vi "ProcessFingers.vi"() -> ()   [LabVIEW 2021]
uses:
  <vilib>/picture/picture.llb/Draw True-Color Pixmap.vi
panel:
  in  "big Or small":i32
  in  "Total Number of Fingers":i32
  in  "range":i32
  out "found fingers":bool
  in  "fingers counter":i32
  out "Little Finger":bool
  out "Ring Finger":bool
  out "Middle Finger":bool
  out "Index Finger":bool
  in  "right counter":i32
  in  "left counter":i32
  in  "j":i32
  in  "i":i32
  in  "bottom counter":i32
  in  "top counter":i32
  in  "thumb counter":i32
  out "Thumb":bool
  out "Right":bool
  out "Left":bool
  out "Black and White Image":picture
  in  "stop":bool
  out "Grayscale Image":picture
  out "Original lmage":picture
  in  "Path":path
  # "Upload Image to be Processed"
  # "Image Data"
  # "Detected Hand"
  # "Detected Fingers"
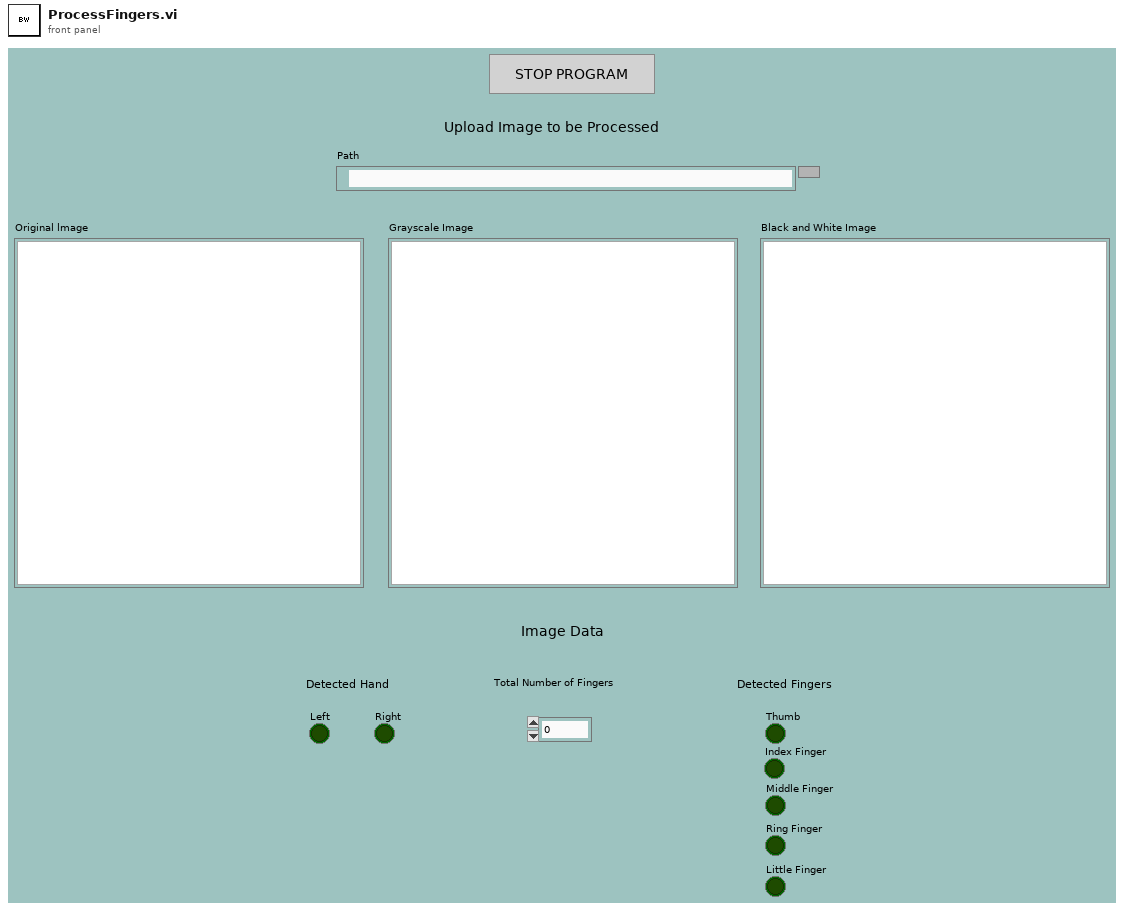
[diagram p1: front panel]
types:
  T1 = typedef "imagedata.ctl" = cluster{"image type":i32, "image depth":i32, "image":u8[], "mask":u8[], "colors":u32[], "Rectangle":cluster{"left":i16, "top":i16, "right":i16, "bottom":i16}}
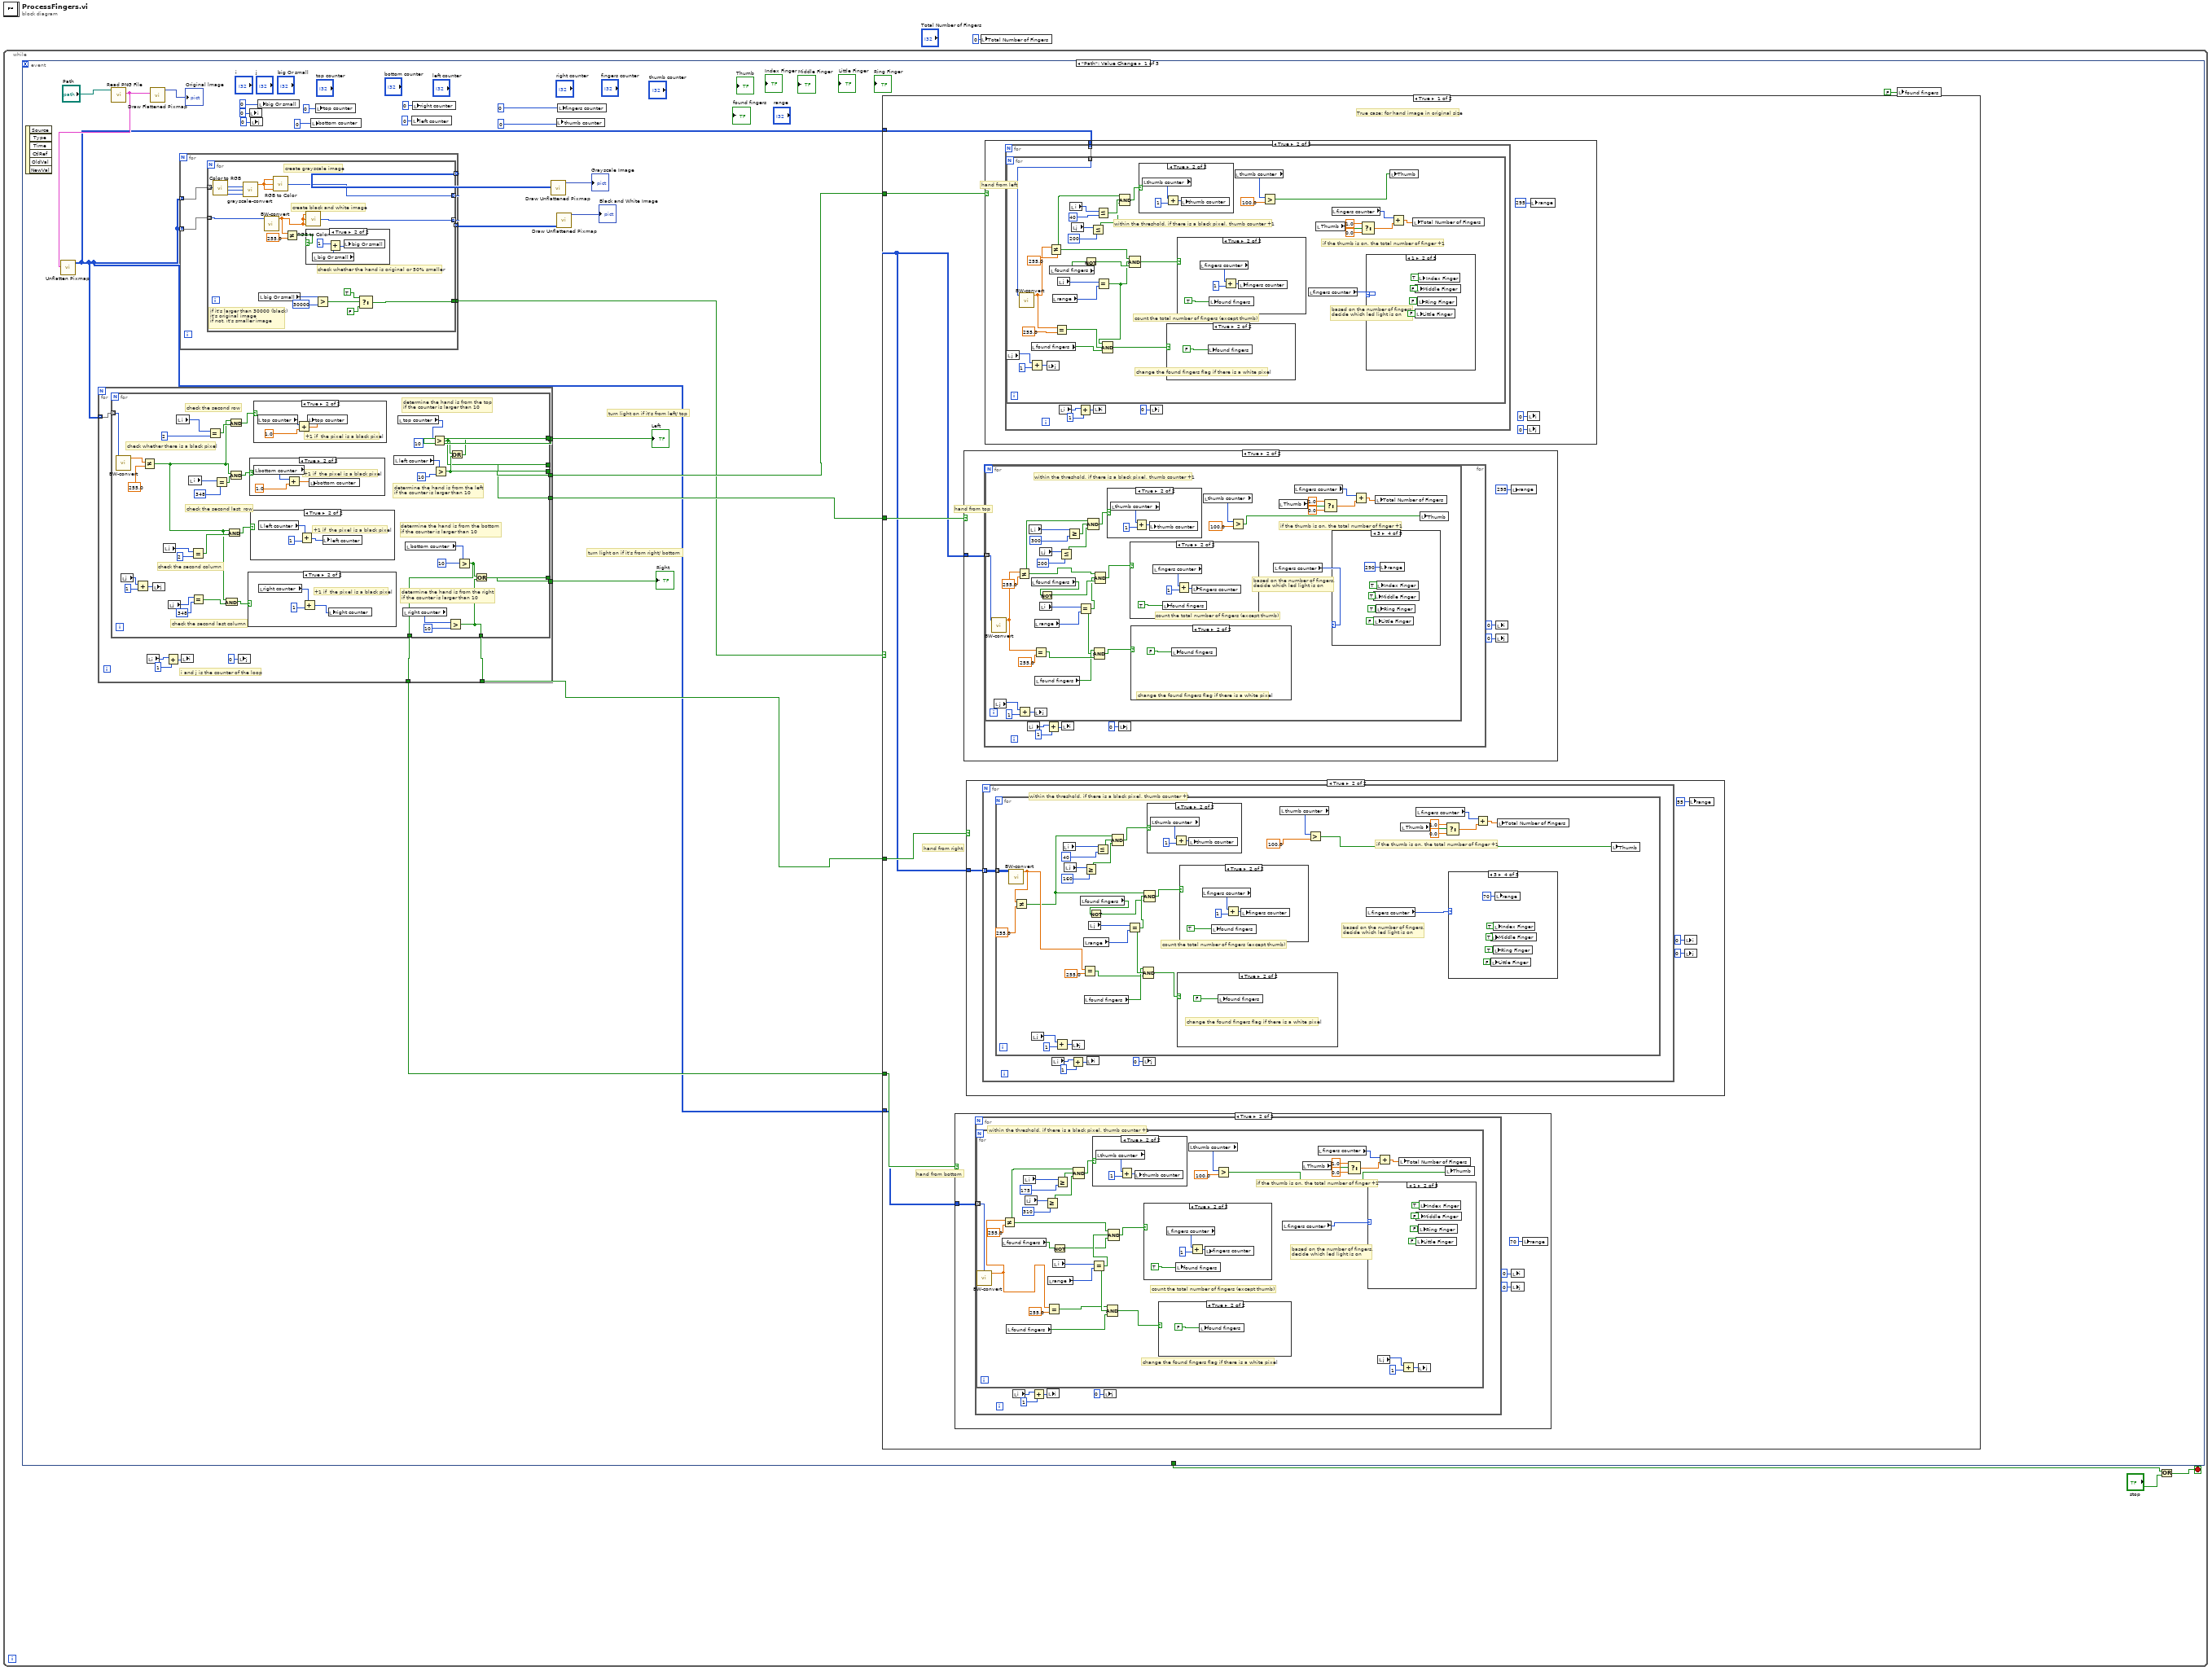
[diagram p0: block diagram]
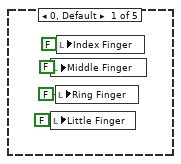
[diagram p5: hidden frame]
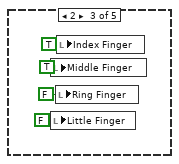
[diagram p6: hidden frame]
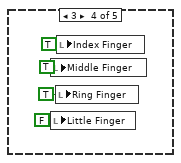
[diagram p7: hidden frame]
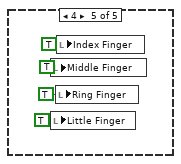
[diagram p8: hidden frame]
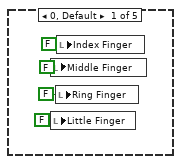
[diagram p11: hidden frame]
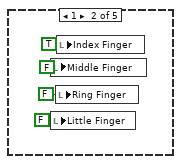
[diagram p12: hidden frame]
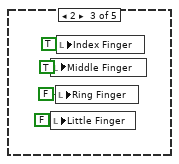
[diagram p13: hidden frame]
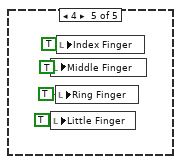
[diagram p14: hidden frame]
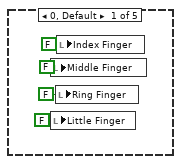
[diagram p19: hidden frame]
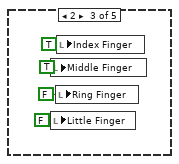
[diagram p20: hidden frame]
diagram:
  n1 = while {
    stop <- w3 stop-if-true
    n2 = event shown="[0] \"Path\": Value Change" {
      selector: _ -> [_ _ _]
      dyn-events: _ -> [_ _ _]
      timeout: _ -> [_ _ _]
      tunnel: [_ TRUE ("x") TRUE ("x")] -> w2
      event "Path": Value Change {
        # "turn light on if it's from left/ top"
        # "turn light on if it's from right/ bottom"
        n3 = event-data() -> ()  [unwired: 1 in, 6 out]
        n4 = call <vilib>:"Read PNG File.vi"("path to PNG file"="Path") -> ("image data"=w27:T1)  [unwired: 8 in, 2 out]
        n5 = call <vilib>:"Unflatten Pixmap.vi"("image data"=w27) -> ("24-bit pixmap"=w6:u32[][])  [unwired: 4 in, 6 out]
        n6 = for {
          tunnel: w6 -> [w625] mode=indexing
          tunnel: [w624] -> w20
          tunnel: [w620] -> w14
          tunnel: [w618] -> w13
          tunnel: [w617] -> w12
          tunnel: [w616] -> w7
          tunnel: [w615] -> w11
          # "i and j is the counter of the loop"
          n7 = for {
            tunnel: w625 -> [w662] mode=indexing
            tunnel: [w645] -> w624
            tunnel: [w630] -> w620
            tunnel: [w629] -> w618
            tunnel: [w628] -> w617
            tunnel: [w627] -> w616
            tunnel: [w626] -> w615
            # "determine the hand is from the right \nif the counter is larger than 10"
            # "determine the hand is from the bottom \nif the counter is larger than 10"
            # "determine the hand is from the left \nif the counter is larger than 10"
            # "determine the hand is from the top \nif the counter is larger than 10"
            # "check the second last column"
            # "check the second last  row"
            # "check the second column"
            # "check the second row"
            # "check whether there is a black pixel"
            n8 = call "BW-convert.vi"("Input pixel"=w662) -> ("Output pixel"=w660:dbl)  [unwired: 10 in]
            n9 = local read "j"() -> (w647:i32)
            n10 = Add(x=w647, y=1) -> (x+y=w657:i32)
            n11 = Not Equal?(x=w660, y=255.0) -> (x != y?=w636:bool)
            n12 = local write "j"(w657) -> ()
            n13 = local read "j"() -> (w644:i32)
            n14 = local read "j"() -> (w638:i32)
            n15 = local read "i"() -> (w655:i32)
            n16 = local read "i"() -> (w650:i32)
            n17 = Equal?(x=w644, y=2) -> (x = y?=w642:bool)
            n18 = Equal?(x=w638, y=348) -> (x = y?=w637:bool)
            n19 = Equal?(x=w655, y=2) -> (x = y?=w653:bool)
            n20 = Equal?(x=w650, y=348) -> (x = y?=w649:bool)
            n21 = Compound Arithmetic op=AND(w636, w637) -> (w635:bool)
            n22 = Compound Arithmetic op=AND(w636, w642) -> (w641:bool)
            n23 = Compound Arithmetic op=AND(w636, w653) -> (w652:bool)
            n24 = Compound Arithmetic op=AND(w636, w649) -> (w648:bool)
            n25 = case shown="True" w635 {
              frame False {
              }
              frame True {
                # "+1 if  the pixel is a black pixel"
                n26 = local read "right counter"() -> (w665:i32)
                n27 = Add(x=w665, y=1) -> (x+y=w664:i32)
                n28 = local write "right counter"(w664) -> ()
              }
            }
            n29 = case shown="True" w648 {
              frame False {
              }
              frame True {
                # "+1 if  the pixel is a black pixel"
                n30 = local read "bottom counter"() -> (w670:i32)
                n31 = Add(x=w670, y=1.0) -> (x+y=w669:dbl)
                n32 = local write "bottom counter"(w669) -> ()
              }
            }
            n33 = case shown="True" w641 {
              frame False {
              }
              frame True {
                # "+1 if  the pixel is a black pixel"
                n34 = local read "left counter"() -> (w668:i32)
                n35 = Add(x=w668, y=1) -> (x+y=w667:i32)
                n36 = local write "left counter"(w667) -> ()
              }
            }
            n37 = case shown="True" w652 {
              frame False {
              }
              frame True {
                # "+1 if  the pixel is a black pixel"
                n38 = local read "top counter"() -> (w673:i32)
                n39 = Add(x=w673, y=1.0) -> (x+y=w674:dbl)
                n40 = local write "top counter"(w674) -> ()
              }
            }
            n41 = local read "left counter"() -> (w640:i32)
            n42 = local read "top counter"() -> (w659:i32)
            n43 = local read "right counter"() -> (w632:i32)
            n44 = local read "bottom counter"() -> (w634:i32)
            n45 = Greater?(x=w659, y=10) -> (0:w628:bool)
            n46 = Greater?(x=w640, y=10) -> (0:w629:bool)
            n47 = Greater?(x=w632, y=10) -> (0:w626:bool)
            n48 = Or(x=w628, y=w629) -> (x .or. y?=w645:bool)
            n49 = Greater?(x=w634, y=10) -> (0:w627:bool)
            n50 = Or(x=w627, y=w626) -> (x .or. y?=w630:bool)
          }
          n51 = local read "i"() -> (w623:i32)
          n52 = Add(x=w623, y=1) -> (x+y=w621:i32)
          n53 = local write "i"(w621) -> ()
          n54 = local write "j"(0 ("j")) -> ()
        }
        "Right" <- w14
        "Left" <- w20
        n55 = call <vilib>:"Draw Flattened Pixmap.vi"("image data"=w27) -> ("new picture"=→"Original lmage":picture)  [unwired: 8 in]
        n56 = for {
          tunnel: w6 -> [w679] mode=indexing
          tunnel: [w678] -> w25 mode=indexing
          tunnel: [w677] -> w23 mode=indexing
          tunnel: w6 -> [w676] mode=indexing
          tunnel: [w675] -> w5
          n57 = for {
            tunnel: w679 -> [w696] mode=indexing
            tunnel: [w695] -> w678 mode=indexing
            tunnel: [w690] -> w677 mode=indexing
            tunnel: w676 -> [w689] mode=indexing
            tunnel: [w680] -> w675
            # "if it's larger than 30000 (black)\nit's original image\nif not, it's smaller image"
            # "check whether the hand is original or 50% smaller"
            # "create black and white image"
            # "create grayscale image"
            n58 = call <vilib>:"Color to RGB.vi"("Color"=w696) -> ("R"=w691:u8, "G"=w694:u8, "B"=w693:u8)  [unwired: 1 out]
            n59 = call "grayscale-convert.vi"("B"=w693, "G"=w694, "R"=w691) -> ("Output pixel"=w692:dbl)  [unwired: 8 in]
            n60 = local read "big Or small"() -> (w684:i32)
            n61 = call "BW-convert.vi"("Input pixel"=w689) -> ("Output pixel"=w688:dbl)  [unwired: 10 in]
            n62 = call <vilib>:"RGB to Color.vi"("B"=w692, "G"=w692, "R"=w692) -> ("Color"=w695:u32)
            n63 = Not Equal?(x=w688, y=255.0) -> (x != y?=w686:bool)
            n64 = call <vilib>:"RGB to Color.vi"("B"=w688, "G"=w688, "R"=w688) -> ("Color"=w690:u32)
            n65 = case shown="True" w686 {
              frame False {
              }
              frame True {
                n66 = local read "big Or small"() -> (w699:i32)
                n67 = Add(x=1, y=w699) -> (x+y=w698:i32)
                n68 = local write "big Or small"(w698) -> ()
              }
            }
            n69 = Greater?(x=w684, y=30000) -> (0:w685:bool)
            n70 = Select(t=TRUE, s=w685, f=FALSE) -> (s? t:f=w680:bool)
          }
        }
        n71 = local write "i"(0 ("i")) -> ()
        n72 = local write "j"(0 ("j")) -> ()
        n73 = local write "big Or small"(0 ("big Or small")) -> ()
        n74 = local write "bottom counter"(0 ("bottom counter")) -> ()
        n75 = local write "top counter"(0 ("counter 2")) -> ()
        n76 = local write "left counter"(0 ("left counter")) -> ()
        n77 = local write "right counter"(0 ("right counter")) -> ()
        n78 = call-poly <vilib>:"Draw Unflattened Pixmap.vi"("data (RGB format)"=w25) -> ("new picture"=→"Grayscale Image":picture)  [unwired: 8 in]
        n79 = local write "thumb counter"(0 ("counter")) -> ()
        n80 = call-poly <vilib>:"Draw Unflattened Pixmap.vi"("data (RGB format)"=w23) -> ("new picture"=→"Black and White Image":picture)  [unwired: 8 in]
        n81 = local write "fingers counter"(0 ("fingers counter")) -> ()
        n82 = case shown="True" w5 {
          tunnel: w13 -> [w35 w328]
          tunnel: w12 -> [w34 w327]
          tunnel: w11 -> [w33 w326]
          tunnel: w6 -> [w32 w325]
          tunnel: w7 -> [w31 w324]
          tunnel: w6 -> [w30 w323]
          frame True {
            # "hand from bottom"
            # "hand from top"
            # "hand from left"
            # "True case: for hand image in original size"
            # "hand from right"
            n83 = case shown="True" w31 {
              tunnel: w30 -> [_ w37]
              frame False {
              }
              frame True {
                n84 = for {
                  tunnel: w37 -> [w40] mode=indexing
                  # "within the threshold, if there is a black pixel, thumb counter +1"
                  n85 = for {
                    tunnel: w40 -> [w68] mode=indexing
                    # "based on the number of fingers,\ndecide which led light is on"
                    # "if the thumb is on, the total number of finger +1"
                    # "change the found fingers flag if there is a white pixel"
                    # "count the total number of fingers (except thumb)"
                    n86 = call "BW-convert.vi"("Input pixel"=w68) -> ("Output pixel"=w46:dbl)  [unwired: 10 in]
                    n87 = local read "found fingers"() -> (w50:bool)
                    n88 = Not Equal?(x=w46, y=255.0) -> (x != y?=w53:bool)
                    n89 = local read "found fingers"() -> (w52:bool)
                    n90 = local read "i"() -> (w65:i32)
                    n91 = local read "j"() -> (w71:i32)
                    n92 = Greater Or Equal?(x=w71, y=310) -> (x >= y?=w69:bool)
                    n93 = Equal?(x=w46, y=255.0) -> (x = y?=w47:bool)
                    n94 = local read "range"() -> (w51:i32)
                    n95 = Not(x=w50) -> (.not. x?=w48:bool)
                    n96 = local read "i"() -> (w54:i32)
                    n97 = Greater Or Equal?(x=w65, y=175) -> (x >= y?=w67:bool)
                    n98 = Compound Arithmetic op=AND(w53, w67, w69) -> (w72:bool)
                    n99 = Equal?(x=w54, y=w51) -> (x = y?=w49:bool)
                    n100 = case shown="True" w72 {
                      frame False {
                      }
                      frame True {
                        n101 = local read "thumb counter"() -> (w106:i32)
                        n102 = Add(x=w106, y=1) -> (x+y=w104:i32)
                        n103 = local write "thumb counter"(w104) -> ()
                      }
                    }
                    n104 = Compound Arithmetic op=AND(w47, w49, w52) -> (w55:bool)
                    n105 = Compound Arithmetic op=AND(w53, w49, w48) -> (w57:bool)
                    n106 = case shown="True" w57 {
                      frame False {
                      }
                      frame True {
                        n107 = local read "fingers counter"() -> (w82:i32)
                        n108 = local write "found fingers"(TRUE ("found fingers")) -> ()
                        n109 = Add(x=w82, y=1) -> (x+y=w81:i32)
                        n110 = local write "fingers counter"(w81) -> ()
                      }
                    }
                    n111 = case shown="True" w55 {
                      frame False {
                      }
                      frame True {
                        n112 = local write "found fingers"(FALSE ("found fingers")) -> ()
                      }
                    }
                    n113 = local read "thumb counter"() -> (w76:i32)
                    n114 = Greater?(x=w76, y=100.0) -> (0:w45:bool)
                    n115 = local read "fingers counter"() -> (w60:i32)
                    n116 = local read "Thumb"() -> (w61:bool)
                    n117 = local read "fingers counter"() -> (w62:i32)
                    n118 = Select(t=1.0, s=w61, f=0.0) -> (s? t:f=w63:dbl)
                    n119 = case shown="1" w60 {
                      frame 0, Default {
                        n120 = local write "Middle Finger"(FALSE ("Thumb 3")) -> ()
                        n121 = local write "Little Finger"(FALSE ("Thumb 5")) -> ()
                        n122 = local write "Ring Finger"(FALSE ("Thumb 4")) -> ()
                        n123 = local write "Index Finger"(FALSE ("Thumb 2")) -> ()
                      }
                      frame 1 {
                        n124 = local write "Middle Finger"(FALSE ("Thumb 3")) -> ()
                        n125 = local write "Little Finger"(FALSE ("Thumb 5")) -> ()
                        n126 = local write "Ring Finger"(FALSE ("Thumb 4")) -> ()
                        n127 = local write "Index Finger"(TRUE ("Thumb 2")) -> ()
                      }
                      frame 2 {
                        n128 = local write "Middle Finger"(TRUE ("Thumb 3")) -> ()
                        n129 = local write "Little Finger"(FALSE ("Thumb 5")) -> ()
                        n130 = local write "Ring Finger"(FALSE ("Thumb 4")) -> ()
                        n131 = local write "Index Finger"(TRUE ("Thumb 2")) -> ()
                      }
                      frame 3 {
                        n132 = local write "Middle Finger"(TRUE ("Thumb 3")) -> ()
                        n133 = local write "Little Finger"(FALSE ("Thumb 5")) -> ()
                        n134 = local write "Ring Finger"(TRUE ("Thumb 4")) -> ()
                        n135 = local write "Index Finger"(TRUE ("Thumb 2")) -> ()
                      }
                      frame 4 {
                        n136 = local write "Middle Finger"(TRUE ("Thumb 3")) -> ()
                        n137 = local write "Little Finger"(TRUE ("Thumb 5")) -> ()
                        n138 = local write "Ring Finger"(TRUE ("Thumb 4")) -> ()
                        n139 = local write "Index Finger"(TRUE ("Thumb 2")) -> ()
                      }
                    }
                    n140 = Add(x=w62, y=w63) -> (x+y=w64:dbl)
                    n141 = local read "j"() -> (w74:i32)
                    n142 = local write "Total Number of Fingers"(w64) -> ()
                    n143 = Add(x=w74, y=1) -> (x+y=w75:i32)
                    n144 = local write "j"(w75) -> ()
                    n145 = local write "Thumb"(w45) -> ()
                  }
                  n146 = local read "i"() -> (w41:i32)
                  n147 = Add(x=w41, y=1) -> (x+y=w43:i32)
                  n148 = local write "i"(w43) -> ()
                  n149 = local write "j"(0 ("j")) -> ()
                }
                n150 = local write "i"(0 ("i")) -> ()
                n151 = local write "j"(0 ("j")) -> ()
                n152 = local write "range"(70 ("range")) -> ()
              }
            }
            n153 = case shown="True" w34 {
              tunnel: w32 -> [_ w108]
              frame False {
              }
              frame True {
                n154 = for {
                  tunnel: w108 -> [w111] mode=indexing
                  n155 = for {
                    tunnel: w111 -> [w139] mode=indexing
                    # "based on the number of fingers,\ndecide which led light is on"
                    # "if the thumb is on, the total number of finger +1"
                    # "change the found fingers flag if there is a white pixel"
                    # "count the total number of fingers (except thumb)"
                    # "within the threshold, if there is a black pixel, thumb counter +1"
                    n156 = call "BW-convert.vi"("Input pixel"=w139) -> ("Output pixel"=w126:dbl)  [unwired: 10 in]
                    n157 = local read "j"() -> (w145:i32)
                    n158 = Not Equal?(x=w126, y=255.0) -> (x != y?=w133:bool)
                    n159 = Add(x=w145, y=1) -> (x+y=w146:i32)
                    n160 = local read "i"() -> (w138:i32)
                    n161 = local read "found fingers"() -> (w132:bool)
                    n162 = Equal?(x=w126, y=255.0) -> (x = y?=w125:bool)
                    n163 = local read "range"() -> (w131:i32)
                    n164 = local write "j"(w146) -> ()
                    n165 = local read "found fingers"() -> (w124:bool)
                    n166 = local read "j"() -> (w142:i32)
                    n167 = Not(x=w132) -> (.not. x?=w134:bool)
                    n168 = local read "i"() -> (w130:i32)
                    n169 = Less Or Equal?(x=w142, y=200) -> (x <= y?=w140:bool)
                    n170 = Greater Or Equal?(x=w138, y=300) -> (x >= y?=w136:bool)
                    n171 = Equal?(x=w130, y=w131) -> (x = y?=w123:bool)
                    n172 = Compound Arithmetic op=AND(w133, w136, w140) -> (w143:bool)
                    n173 = Compound Arithmetic op=AND(w124, w123, w125) -> (w128:bool)
                    n174 = Compound Arithmetic op=AND(w133, w123, w134) -> (w129:bool)
                    n175 = case shown="True" w143 {
                      frame False {
                      }
                      frame True {
                        n176 = local read "thumb counter"() -> (w178:i32)
                        n177 = Add(x=w178, y=1) -> (x+y=w176:i32)
                        n178 = local write "thumb counter"(w176) -> ()
                      }
                    }
                    n179 = case shown="True" w129 {
                      frame False {
                      }
                      frame True {
                        n180 = local read "fingers counter"() -> (w174:i32)
                        n181 = local write "found fingers"(TRUE ("found fingers")) -> ()
                        n182 = Add(x=w174, y=1) -> (x+y=w173:i32)
                        n183 = local write "fingers counter"(w173) -> ()
                      }
                    }
                    n184 = case shown="True" w128 {
                      frame False {
                      }
                      frame True {
                        n185 = local write "found fingers"(FALSE ("found fingers")) -> ()
                      }
                    }
                    n186 = local read "thumb counter"() -> (w147:i32)
                    n187 = Greater?(x=w147, y=100.0) -> (0:w116:bool)
                    n188 = local read "fingers counter"() -> (w135:i32)
                    n189 = local read "Thumb"() -> (w117:bool)
                    n190 = local read "fingers counter"() -> (w120:i32)
                    n191 = Select(t=1.0, s=w117, f=0.0) -> (s? t:f=w121:dbl)
                    n192 = case shown="3" w135 {
                      frame 0, Default {
                        n193 = local write "Middle Finger"(FALSE ("Thumb 3")) -> ()
                        n194 = local write "Little Finger"(FALSE ("Thumb 5")) -> ()
                        n195 = local write "Ring Finger"(FALSE ("Thumb 4")) -> ()
                        n196 = local write "Index Finger"(FALSE ("Thumb 2")) -> ()
                      }
                      frame 1 {
                        n197 = local write "Middle Finger"(FALSE ("Thumb 3")) -> ()
                        n198 = local write "Little Finger"(FALSE ("Thumb 5")) -> ()
                        n199 = local write "Ring Finger"(FALSE ("Thumb 4")) -> ()
                        n200 = local write "Index Finger"(TRUE ("Thumb 2")) -> ()
                      }
                      frame 2 {
                        n201 = local write "Middle Finger"(TRUE ("Thumb 3")) -> ()
                        n202 = local write "Little Finger"(FALSE ("Thumb 5")) -> ()
                        n203 = local write "Ring Finger"(FALSE ("Thumb 4")) -> ()
                        n204 = local write "Index Finger"(TRUE ("Thumb 2")) -> ()
                      }
                      frame 3 {
                        n205 = local write "Middle Finger"(TRUE ("Thumb 3")) -> ()
                        n206 = local write "Little Finger"(FALSE ("Thumb 5")) -> ()
                        n207 = local write "Ring Finger"(TRUE ("Thumb 4")) -> ()
                        n208 = local write "Index Finger"(TRUE ("Thumb 2")) -> ()
                        n209 = local write "range"(290 ("range")) -> ()
                      }
                      frame 4 {
                        n210 = local write "Middle Finger"(TRUE ("Thumb 3")) -> ()
                        n211 = local write "Little Finger"(TRUE ("Thumb 5")) -> ()
                        n212 = local write "Ring Finger"(TRUE ("Thumb 4")) -> ()
                        n213 = local write "Index Finger"(TRUE ("Thumb 2")) -> ()
                      }
                    }
                    n214 = Add(x=w120, y=w121) -> (x+y=w122:dbl)
                    n215 = local write "Total Number of Fingers"(w122) -> ()
                    n216 = local write "Thumb"(w116) -> ()
                  }
                  n217 = local read "i"() -> (w112:i32)
                  n218 = Add(x=w112, y=1) -> (x+y=w114:i32)
                  n219 = local write "i"(w114) -> ()
                  n220 = local write "j"(0 ("j")) -> ()
                }
                n221 = local write "i"(0 ("i")) -> ()
                n222 = local write "j"(0 ("j")) -> ()
                n223 = local write "range"(295 ("range")) -> ()
              }
            }
            n224 = case shown="True" w33 {
              tunnel: w32 -> [_ w252]
              frame False {
              }
              frame True {
                n225 = for {
                  tunnel: w252 -> [w255] mode=indexing
                  # "within the threshold, if there is a black pixel, thumb counter +1"
                  n226 = for {
                    tunnel: w255 -> [w283] mode=indexing
                    # "based on the number of fingers,\ndecide which led light is on"
                    # "if the thumb is on, the total number of finger +1"
                    # "count the total number of fingers (except thumb)"
                    n227 = call "BW-convert.vi"("Input pixel"=w283) -> ("Output pixel"=w264:dbl)  [unwired: 10 in]
                    n228 = Not Equal?(x=w264, y=255.0) -> (x != y?=w261:bool)
                    n229 = local read "j"() -> (w289:i32)
                    n230 = Add(x=w289, y=1) -> (x+y=w290:i32)
                    n231 = local read "i"() -> (w282:i32)
                    n232 = local read "j"() -> (w286:i32)
                    n233 = local write "j"(w290) -> ()
                    n234 = local read "found fingers"() -> (w263:bool)
                    n235 = Equal?(x=w264, y=255.0) -> (x = y?=w270:bool)
                    n236 = Greater Or Equal?(x=w286, y=160) -> (x >= y?=w284:bool)
                    n237 = local read "range"() -> (w268:i32)
                    n238 = local read "found fingers"() -> (w271:bool)
                    n239 = Not(x=w263) -> (.not. x?=w267:bool)
                    n240 = local read "j"() -> (w269:i32)
                    n241 = Less Or Equal?(x=w282, y=40) -> (x <= y?=w280:bool)
                    n242 = Compound Arithmetic op=AND(w261, w280, w284) -> (w287:bool)
                    n243 = Equal?(x=w269, y=w268) -> (x = y?=w272:bool)
                    n244 = Compound Arithmetic op=AND(w271, w272, w270) -> (w266:bool)
                    n245 = Compound Arithmetic op=AND(w261, w272, w267) -> (w262:bool)
                    n246 = case shown="True" w287 {
                      frame False {
                      }
                      frame True {
                        n247 = local read "thumb counter"() -> (w322:i32)
                        n248 = Add(x=w322, y=1) -> (x+y=w320:i32)
                        n249 = local write "thumb counter"(w320) -> ()
                      }
                    }
                    n250 = case shown="True" w266 {
                      frame False {
                      }
                      frame True {
                        # "change the found fingers flag if there is a white pixel"
                        n251 = local write "found fingers"(FALSE ("found fingers")) -> ()
                      }
                    }
                    n252 = case shown="True" w262 {
                      frame False {
                      }
                      frame True {
                        n253 = local read "fingers counter"() -> (w297:i32)
                        n254 = local write "found fingers"(TRUE ("found fingers")) -> ()
                        n255 = Add(x=w297, y=1) -> (x+y=w296:i32)
                        n256 = local write "fingers counter"(w296) -> ()
                      }
                    }
                    n257 = local read "thumb counter"() -> (w291:i32)
                    n258 = Greater?(x=w291, y=100.0) -> (0:w260:bool)
                    n259 = local read "fingers counter"() -> (w279:i32)
                    n260 = local read "Thumb"() -> (w278:bool)
                    n261 = local read "fingers counter"() -> (w275:i32)
                    n262 = Select(t=1.0, s=w278, f=0.0) -> (s? t:f=w274:dbl)
                    n263 = case shown="3" w279 {
                      frame 0, Default {
                        n264 = local write "Middle Finger"(FALSE ("Thumb 3")) -> ()
                        n265 = local write "Little Finger"(FALSE ("Thumb 5")) -> ()
                        n266 = local write "Ring Finger"(FALSE ("Thumb 4")) -> ()
                        n267 = local write "Index Finger"(FALSE ("Thumb 2")) -> ()
                      }
                      frame 1 {
                        n268 = local write "Middle Finger"(FALSE ("Thumb 3")) -> ()
                        n269 = local write "Little Finger"(FALSE ("Thumb 5")) -> ()
                        n270 = local write "Ring Finger"(FALSE ("Thumb 4")) -> ()
                        n271 = local write "Index Finger"(TRUE ("Thumb 2")) -> ()
                      }
                      frame 2 {
                        n272 = local write "Middle Finger"(TRUE ("Thumb 3")) -> ()
                        n273 = local write "Little Finger"(FALSE ("Thumb 5")) -> ()
                        n274 = local write "Ring Finger"(FALSE ("Thumb 4")) -> ()
                        n275 = local write "Index Finger"(TRUE ("Thumb 2")) -> ()
                      }
                      frame 3 {
                        n276 = local write "Middle Finger"(TRUE ("Thumb 3")) -> ()
                        n277 = local write "Little Finger"(FALSE ("Thumb 5")) -> ()
                        n278 = local write "Ring Finger"(TRUE ("Thumb 4")) -> ()
                        n279 = local write "Index Finger"(TRUE ("Thumb 2")) -> ()
                        n280 = local write "range"(70 ("range")) -> ()
                      }
                      frame 4 {
                        n281 = local write "Middle Finger"(TRUE ("Thumb 3")) -> ()
                        n282 = local write "Little Finger"(TRUE ("Thumb 5")) -> ()
                        n283 = local write "Ring Finger"(TRUE ("Thumb 4")) -> ()
                        n284 = local write "Index Finger"(TRUE ("Thumb 2")) -> ()
                      }
                    }
                    n285 = Add(x=w275, y=w274) -> (x+y=w273:dbl)
                    n286 = local write "Total Number of Fingers"(w273) -> ()
                    n287 = local write "Thumb"(w260) -> ()
                  }
                  n288 = local read "i"() -> (w256:i32)
                  n289 = Add(x=w256, y=1) -> (x+y=w258:i32)
                  n290 = local write "i"(w258) -> ()
                  n291 = local write "j"(0 ("j")) -> ()
                }
                n292 = local write "i"(0 ("i")) -> ()
                n293 = local write "j"(0 ("j")) -> ()
                n294 = local write "range"(55 ("range")) -> ()
              }
            }
            n295 = case shown="True" w35 {
              tunnel: w32 -> [_ w182]
              frame False {
              }
              frame True {
                n296 = for {
                  tunnel: w182 -> [w187] mode=indexing
                  n297 = for {
                    tunnel: w187 -> [w220] mode=indexing
                    # "based on the number of fingers,\ndecide which led light is on"
                    # "if the thumb is on, the total number of finger +1"
                    # "change the found fingers flag if there is a white pixel"
                    # "count the total number of fingers (except thumb)"
                    # "within the threshold, if there is a black pixel, thumb counter +1"
                    n298 = local read "j"() -> (w216:i32)
                    n299 = call "BW-convert.vi"("Input pixel"=w220) -> ("Output pixel"=w202:dbl)  [unwired: 10 in]
                    n300 = Add(x=w216, y=1) -> (x+y=w217:i32)
                    n301 = local read "found fingers"() -> (w198:bool)
                    n302 = local write "j"(w217) -> ()
                    n303 = Not Equal?(x=w202, y=255.0) -> (x != y?=w206:bool)
                    n304 = local read "found fingers"() -> (w204:bool)
                    n305 = local read "range"() -> (w195:i32)
                    n306 = Equal?(x=w202, y=255.0) -> (x = y?=w199:bool)
                    n307 = local read "j"() -> (w207:i32)
                    n308 = local read "i"() -> (w213:i32)
                    n309 = local read "j"() -> (w210:i32)
                    n310 = Not(x=w204) -> (.not. x?=w203:bool)
                    n311 = Less Or Equal?(x=w210, y=200) -> (x <= y?=w208:bool)
                    n312 = Less Or Equal?(x=w213, y=40) -> (x <= y?=w211:bool)
                    n313 = Equal?(x=w207, y=w195) -> (x = y?=w200:bool)
                    n314 = Compound Arithmetic op=AND(w200, w199, w198) -> (w197:bool)
                    n315 = Compound Arithmetic op=AND(w206, w211, w208) -> (w214:bool)
                    n316 = Compound Arithmetic op=AND(w206, w200, w203) -> (w205:bool)
                    n317 = case shown="True" w214 {
                      frame False {
                      }
                      frame True {
                        n318 = local read "thumb counter"() -> (w250:i32)
                        n319 = Add(x=w250, y=1) -> (x+y=w248:i32)
                        n320 = local write "thumb counter"(w248) -> ()
                      }
                    }
                    n321 = case shown="True" w197 {
                      frame False {
                      }
                      frame True {
                        n322 = local write "found fingers"(FALSE ("found fingers")) -> ()
                      }
                    }
                    n323 = case shown="True" w205 {
                      frame False {
                      }
                      frame True {
                        n324 = local read "fingers counter"() -> (w246:i32)
                        n325 = local write "found fingers"(TRUE ("found fingers")) -> ()
                        n326 = Add(x=w246, y=1) -> (x+y=w245:i32)
                        n327 = local write "fingers counter"(w245) -> ()
                      }
                    }
                    n328 = local read "thumb counter"() -> (w218:i32)
                    n329 = Greater?(x=w218, y=100.0) -> (0:w196:bool)
                    n330 = local read "fingers counter"() -> (w194:i32)
                    n331 = local read "Thumb"() -> (w193:bool)
                    n332 = local read "fingers counter"() -> (w190:i32)
                    n333 = Select(t=1.0, s=w193, f=0.0) -> (s? t:f=w189:dbl)
                    n334 = case shown="1" w194 {
                      frame 0, Default {
                        n335 = local write "Middle Finger"(FALSE ("Thumb 3")) -> ()
                        n336 = local write "Little Finger"(FALSE ("Thumb 5")) -> ()
                        n337 = local write "Ring Finger"(FALSE ("Thumb 4")) -> ()
                        n338 = local write "Index Finger"(FALSE ("Thumb 2")) -> ()
                      }
                      frame 1 {
                        n339 = local write "Middle Finger"(FALSE ("Thumb 3")) -> ()
                        n340 = local write "Little Finger"(FALSE ("Thumb 5")) -> ()
                        n341 = local write "Ring Finger"(FALSE ("Thumb 4")) -> ()
                        n342 = local write "Index Finger"(TRUE ("Thumb 2")) -> ()
                      }
                      frame 2 {
                        n343 = local write "Middle Finger"(TRUE ("Thumb 3")) -> ()
                        n344 = local write "Little Finger"(FALSE ("Thumb 5")) -> ()
                        n345 = local write "Ring Finger"(FALSE ("Thumb 4")) -> ()
                        n346 = local write "Index Finger"(TRUE ("Thumb 2")) -> ()
                      }
                      frame 3 {
                        n347 = local write "Middle Finger"(TRUE ("Thumb 3")) -> ()
                        n348 = local write "Little Finger"(FALSE ("Thumb 5")) -> ()
                        n349 = local write "Ring Finger"(TRUE ("Thumb 4")) -> ()
                        n350 = local write "Index Finger"(TRUE ("Thumb 2")) -> ()
                        n351 = local write "range"(290 ("range")) -> ()
                      }
                      frame 4 {
                        n352 = local write "Middle Finger"(TRUE ("Thumb 3")) -> ()
                        n353 = local write "Little Finger"(TRUE ("Thumb 5")) -> ()
                        n354 = local write "Ring Finger"(TRUE ("Thumb 4")) -> ()
                        n355 = local write "Index Finger"(TRUE ("Thumb 2")) -> ()
                      }
                    }
                    n356 = local write "Thumb"(w196) -> ()
                    n357 = Add(x=w190, y=w189) -> (x+y=w188:dbl)
                    n358 = local write "Total Number of Fingers"(w188) -> ()
                  }
                  n359 = local read "i"() -> (w183:i32)
                  n360 = Add(x=w183, y=1) -> (x+y=w185:i32)
                  n361 = local write "i"(w185) -> ()
                  n362 = local write "j"(0 ("j")) -> ()
                }
                n363 = local write "i"(0 ("i")) -> ()
                n364 = local write "j"(0 ("j")) -> ()
                n365 = local write "range"(295 ("range")) -> ()
              }
            }
          }
          frame False {
            # "False case: for 50% smaller hand image"
            # "hand from left"
            n366 = case shown="True" w326 {
              tunnel: w325 -> [_ w544]
              frame False {
              }
              frame True {
                n367 = for {
                  tunnel: w544 -> [w547] mode=indexing
                  # "within the threshold, if there is a black pixel, thumb counter +1"
                  n368 = for {
                    tunnel: w547 -> [w575] mode=indexing
                    # "based on the number of fingers,\ndecide which led light is on"
                    # "if the thumb is on, the total number of finger +1"
                    # "hand from right"
                    n369 = call "BW-convert.vi"("Input pixel"=w575) -> ("Output pixel"=w556:dbl)  [unwired: 10 in]
                    n370 = Not Equal?(x=w556, y=255.0) -> (x != y?=w553:bool)
                    n371 = local read "j"() -> (w581:i32)
                    n372 = Add(x=w581, y=1) -> (x+y=w582:i32)
                    n373 = local read "i"() -> (w574:i32)
                    n374 = local read "j"() -> (w578:i32)
                    n375 = local write "j"(w582) -> ()
                    n376 = local read "found fingers"() -> (w555:bool)
                    n377 = Equal?(x=w556, y=255.0) -> (x = y?=w562:bool)
                    n378 = Greater Or Equal?(x=w578, y=150) -> (x >= y?=w576:bool)
                    n379 = local read "range"() -> (w560:i32)
                    n380 = local read "found fingers"() -> (w563:bool)
                    n381 = Not(x=w555) -> (.not. x?=w559:bool)
                    n382 = local read "j"() -> (w561:i32)
                    n383 = Less Or Equal?(x=w574, y=130) -> (x <= y?=w572:bool)
                    n384 = Compound Arithmetic op=AND(w553, w572, w576) -> (w579:bool)
                    n385 = Equal?(x=w561, y=w560) -> (x = y?=w564:bool)
                    n386 = Compound Arithmetic op=AND(w563, w564, w562) -> (w558:bool)
                    n387 = Compound Arithmetic op=AND(w553, w564, w559) -> (w554:bool)
                    n388 = case shown="True" w579 {
                      frame False {
                      }
                      frame True {
                        n389 = local read "thumb counter"() -> (w614:i32)
                        n390 = Add(x=w614, y=1) -> (x+y=w612:i32)
                        n391 = local write "thumb counter"(w612) -> ()
                      }
                    }
                    n392 = case shown="True" w554 {
                      frame False {
                      }
                      frame True {
                        # "count the total number of fingers (except thumb)"
                        n393 = local read "fingers counter"() -> (w589:i32)
                        n394 = local write "found fingers"(TRUE ("found fingers")) -> ()
                        n395 = Add(x=w589, y=1) -> (x+y=w588:i32)
                        n396 = local write "fingers counter"(w588) -> ()
                      }
                    }
                    n397 = case shown="True" w558 {
                      frame False {
                      }
                      frame True {
                        # "change the found fingers flag if there is a white pixel"
                        n398 = local write "found fingers"(FALSE ("found fingers")) -> ()
                      }
                    }
                    n399 = local read "thumb counter"() -> (w583:i32)
                    n400 = Greater?(x=w583, y=100.0) -> (0:w552:bool)
                    n401 = local read "fingers counter"() -> (w571:i32)
                    n402 = local read "Thumb"() -> (w570:bool)
                    n403 = local read "fingers counter"() -> (w567:i32)
                    n404 = Select(t=1.0, s=w570, f=0.0) -> (s? t:f=w566:dbl)
                    n405 = case shown="3" w571 {
                      frame 0, Default {
                        n406 = local write "Middle Finger"(FALSE ("Thumb 3")) -> ()
                        n407 = local write "Little Finger"(FALSE ("Thumb 5")) -> ()
                        n408 = local write "Ring Finger"(FALSE ("Thumb 4")) -> ()
                        n409 = local write "Index Finger"(FALSE ("Thumb 2")) -> ()
                      }
                      frame 1 {
                        n410 = local write "Middle Finger"(FALSE ("Thumb 3")) -> ()
                        n411 = local write "Little Finger"(FALSE ("Thumb 5")) -> ()
                        n412 = local write "Ring Finger"(FALSE ("Thumb 4")) -> ()
                        n413 = local write "Index Finger"(TRUE ("Thumb 2")) -> ()
                      }
                      frame 2 {
                        n414 = local write "Middle Finger"(TRUE ("Thumb 3")) -> ()
                        n415 = local write "Little Finger"(FALSE ("Thumb 5")) -> ()
                        n416 = local write "Ring Finger"(FALSE ("Thumb 4")) -> ()
                        n417 = local write "Index Finger"(TRUE ("Thumb 2")) -> ()
                      }
                      frame 3 {
                        n418 = local write "Middle Finger"(TRUE ("Thumb 3")) -> ()
                        n419 = local write "Little Finger"(FALSE ("Thumb 5")) -> ()
                        n420 = local write "Ring Finger"(TRUE ("Thumb 4")) -> ()
                        n421 = local write "Index Finger"(TRUE ("Thumb 2")) -> ()
                        n422 = local write "range"(110 ("range")) -> ()
                      }
                      frame 4 {
                        n423 = local write "Middle Finger"(TRUE ("Thumb 3")) -> ()
                        n424 = local write "Little Finger"(TRUE ("Thumb 5")) -> ()
                        n425 = local write "Ring Finger"(TRUE ("Thumb 4")) -> ()
                        n426 = local write "Index Finger"(TRUE ("Thumb 2")) -> ()
                      }
                    }
                    n427 = Add(x=w567, y=w566) -> (x+y=w565:dbl)
                    n428 = local write "Total Number of Fingers"(w565) -> ()
                    n429 = local write "Thumb"(w552) -> ()
                  }
                  n430 = local read "i"() -> (w548:i32)
                  n431 = Add(x=w548, y=1) -> (x+y=w550:i32)
                  n432 = local write "i"(w550) -> ()
                  n433 = local write "j"(0 ("j")) -> ()
                }
                n434 = local write "i"(0 ("i")) -> ()
                n435 = local write "j"(0 ("j")) -> ()
                n436 = local write "range"(90 ("range")) -> ()
              }
            }
            n437 = case shown="True" w324 {
              tunnel: w323 -> [_ w330]
              frame False {
              }
              frame True {
                n438 = for {
                  tunnel: w330 -> [w333] mode=indexing
                  # "within the threshold, if there is a black pixel, thumb counter +1"
                  # "hand from bottom"
                  n439 = for {
                    tunnel: w333 -> [w361] mode=indexing
                    # "based on the number of fingers,\ndecide which led light is on"
                    # "if the thumb is on, the total number of finger +1"
                    n440 = call "BW-convert.vi"("Input pixel"=w361) -> ("Output pixel"=w339:dbl)  [unwired: 10 in]
                    n441 = local read "found fingers"() -> (w343:bool)
                    n442 = Not Equal?(x=w339, y=255.0) -> (x != y?=w346:bool)
                    n443 = local read "found fingers"() -> (w345:bool)
                    n444 = local read "i"() -> (w358:i32)
                    n445 = local read "j"() -> (w364:i32)
                    n446 = Greater Or Equal?(x=w364, y=230) -> (x >= y?=w362:bool)
                    n447 = Equal?(x=w339, y=255.0) -> (x = y?=w340:bool)
                    n448 = local read "range"() -> (w344:i32)
                    n449 = Not(x=w343) -> (.not. x?=w341:bool)
                    n450 = local read "i"() -> (w347:i32)
                    n451 = Greater Or Equal?(x=w358, y=175) -> (x >= y?=w360:bool)
                    n452 = Compound Arithmetic op=AND(w346, w360, w362) -> (w365:bool)
                    n453 = Equal?(x=w347, y=w344) -> (x = y?=w342:bool)
                    n454 = case shown="True" w365 {
                      frame False {
                      }
                      frame True {
                        n455 = local read "thumb counter"() -> (w399:i32)
                        n456 = Add(x=w399, y=1) -> (x+y=w397:i32)
                        n457 = local write "thumb counter"(w397) -> ()
                      }
                    }
                    n458 = Compound Arithmetic op=AND(w340, w342, w345) -> (w348:bool)
                    n459 = Compound Arithmetic op=AND(w346, w342, w341) -> (w350:bool)
                    n460 = case shown="True" w350 {
                      frame False {
                      }
                      frame True {
                        # "count the total number of fingers (except thumb)"
                        n461 = local read "fingers counter"() -> (w375:i32)
                        n462 = local write "found fingers"(TRUE ("found fingers")) -> ()
                        n463 = Add(x=w375, y=1) -> (x+y=w374:i32)
                        n464 = local write "fingers counter"(w374) -> ()
                      }
                    }
                    n465 = case shown="True" w348 {
                      frame False {
                      }
                      frame True {
                        # "change the found fingers flag if there is a white pixel"
                        n466 = local write "found fingers"(FALSE ("found fingers")) -> ()
                      }
                    }
                    n467 = local read "thumb counter"() -> (w369:i32)
                    n468 = Greater?(x=w369, y=100.0) -> (0:w338:bool)
                    n469 = local read "fingers counter"() -> (w353:i32)
                    n470 = local read "Thumb"() -> (w354:bool)
                    n471 = local read "fingers counter"() -> (w355:i32)
                    n472 = Select(t=1.0, s=w354, f=0.0) -> (s? t:f=w356:dbl)
                    n473 = case shown="3" w353 {
                      frame 0, Default {
                        n474 = local write "Middle Finger"(FALSE ("Thumb 3")) -> ()
                        n475 = local write "Little Finger"(FALSE ("Thumb 5")) -> ()
                        n476 = local write "Ring Finger"(FALSE ("Thumb 4")) -> ()
                        n477 = local write "Index Finger"(FALSE ("Thumb 2")) -> ()
                      }
                      frame 1 {
                        n478 = local write "Middle Finger"(FALSE ("Thumb 3")) -> ()
                        n479 = local write "Little Finger"(FALSE ("Thumb 5")) -> ()
                        n480 = local write "Ring Finger"(FALSE ("Thumb 4")) -> ()
                        n481 = local write "Index Finger"(TRUE ("Thumb 2")) -> ()
                      }
                      frame 2 {
                        n482 = local write "Middle Finger"(TRUE ("Thumb 3")) -> ()
                        n483 = local write "Little Finger"(FALSE ("Thumb 5")) -> ()
                        n484 = local write "Ring Finger"(FALSE ("Thumb 4")) -> ()
                        n485 = local write "Index Finger"(TRUE ("Thumb 2")) -> ()
                      }
                      frame 3 {
                        n486 = local write "Middle Finger"(TRUE ("Thumb 3")) -> ()
                        n487 = local write "Little Finger"(FALSE ("Thumb 5")) -> ()
                        n488 = local write "Ring Finger"(TRUE ("Thumb 4")) -> ()
                        n489 = local write "Index Finger"(TRUE ("Thumb 2")) -> ()
                      }
                      frame 4 {
                        n490 = local write "Middle Finger"(TRUE ("Thumb 3")) -> ()
                        n491 = local write "Little Finger"(TRUE ("Thumb 5")) -> ()
                        n492 = local write "Ring Finger"(TRUE ("Thumb 4")) -> ()
                        n493 = local write "Index Finger"(TRUE ("Thumb 2")) -> ()
                      }
                    }
                    n494 = Add(x=w355, y=w356) -> (x+y=w357:dbl)
                    n495 = local read "j"() -> (w367:i32)
                    n496 = local write "Total Number of Fingers"(w357) -> ()
                    n497 = Add(x=w367, y=1) -> (x+y=w368:i32)
                    n498 = local write "j"(w368) -> ()
                    n499 = local write "Thumb"(w338) -> ()
                  }
                  n500 = local read "i"() -> (w334:i32)
                  n501 = Add(x=w334, y=1) -> (x+y=w336:i32)
                  n502 = local write "i"(w336) -> ()
                  n503 = local write "j"(0 ("j")) -> ()
                }
                n504 = local write "i"(0 ("i")) -> ()
                n505 = local write "j"(0 ("j")) -> ()
                n506 = local write "range"(110 ("range")) -> ()
              }
            }
            n507 = case shown="True" w327 {
              tunnel: w325 -> [_ w401]
              frame False {
              }
              frame True {
                # "hand from top"
                n508 = for {
                  tunnel: w401 -> [w404] mode=indexing
                  n509 = for {
                    tunnel: w404 -> [w432] mode=indexing
                    # "based on the number of fingers,\ndecide which led light is on"
                    # "if the thumb is on, the total number of finger +1"
                    # "within the threshold, if there is a black pixel, thumb counter +1"
                    n510 = call "BW-convert.vi"("Input pixel"=w432) -> ("Output pixel"=w419:dbl)  [unwired: 10 in]
                    n511 = local read "j"() -> (w438:i32)
                    n512 = Not Equal?(x=w419, y=255.0) -> (x != y?=w426:bool)
                    n513 = Add(x=w438, y=1) -> (x+y=w439:i32)
                    n514 = local read "i"() -> (w431:i32)
                    n515 = local read "found fingers"() -> (w425:bool)
                    n516 = Equal?(x=w419, y=255.0) -> (x = y?=w418:bool)
                    n517 = local read "range"() -> (w424:i32)
                    n518 = local write "j"(w439) -> ()
                    n519 = local read "found fingers"() -> (w417:bool)
                    n520 = local read "j"() -> (w435:i32)
                    n521 = Not(x=w425) -> (.not. x?=w427:bool)
                    n522 = local read "i"() -> (w423:i32)
                    n523 = Greater Or Equal?(x=w435, y=280) -> (x >= y?=w433:bool)
                    n524 = Less Or Equal?(x=w431, y=190) -> (x <= y?=w429:bool)
                    n525 = Equal?(x=w423, y=w424) -> (x = y?=w416:bool)
                    n526 = Compound Arithmetic op=AND(w426, w429, w433) -> (w436:bool)
                    n527 = Compound Arithmetic op=AND(w417, w416, w418) -> (w421:bool)
                    n528 = Compound Arithmetic op=AND(w426, w416, w427) -> (w422:bool)
                    n529 = case shown="True" w436 {
                      frame False {
                      }
                      frame True {
                        n530 = local read "thumb counter"() -> (w470:i32)
                        n531 = Add(x=w470, y=1) -> (x+y=w468:i32)
                        n532 = local write "thumb counter"(w468) -> ()
                      }
                    }
                    n533 = case shown="True" w422 {
                      frame False {
                      }
                      frame True {
                        # "count the total number of fingers (except thumb)"
                        n534 = local read "fingers counter"() -> (w466:i32)
                        n535 = local write "found fingers"(TRUE ("found fingers")) -> ()
                        n536 = Add(x=w466, y=1) -> (x+y=w465:i32)
                        n537 = local write "fingers counter"(w465) -> ()
                      }
                    }
                    n538 = case shown="True" w421 {
                      frame False {
                      }
                      frame True {
                        # "change the found fingers flag if there is a white pixel"
                        n539 = local write "found fingers"(FALSE ("found fingers")) -> ()
                      }
                    }
                    n540 = local read "thumb counter"() -> (w440:i32)
                    n541 = Greater?(x=w440, y=100.0) -> (0:w409:bool)
                    n542 = local read "fingers counter"() -> (w428:i32)
                    n543 = local read "Thumb"() -> (w410:bool)
                    n544 = local read "fingers counter"() -> (w413:i32)
                    n545 = Select(t=1.0, s=w410, f=0.0) -> (s? t:f=w414:dbl)
                    n546 = case shown="3" w428 {
                      frame 0, Default {
                        n547 = local write "Middle Finger"(FALSE ("Thumb 3")) -> ()
                        n548 = local write "Little Finger"(FALSE ("Thumb 5")) -> ()
                        n549 = local write "Ring Finger"(FALSE ("Thumb 4")) -> ()
                        n550 = local write "Index Finger"(FALSE ("Thumb 2")) -> ()
                      }
                      frame 1 {
                        n551 = local write "Middle Finger"(FALSE ("Thumb 3")) -> ()
                        n552 = local write "Little Finger"(FALSE ("Thumb 5")) -> ()
                        n553 = local write "Ring Finger"(FALSE ("Thumb 4")) -> ()
                        n554 = local write "Index Finger"(TRUE ("Thumb 2")) -> ()
                      }
                      frame 2 {
                        n555 = local write "Middle Finger"(TRUE ("Thumb 3")) -> ()
                        n556 = local write "Little Finger"(FALSE ("Thumb 5")) -> ()
                        n557 = local write "Ring Finger"(FALSE ("Thumb 4")) -> ()
                        n558 = local write "Index Finger"(TRUE ("Thumb 2")) -> ()
                      }
                      frame 3 {
                        n559 = local write "Middle Finger"(TRUE ("Thumb 3")) -> ()
                        n560 = local write "Little Finger"(FALSE ("Thumb 5")) -> ()
                        n561 = local write "Ring Finger"(TRUE ("Thumb 4")) -> ()
                        n562 = local write "Index Finger"(TRUE ("Thumb 2")) -> ()
                      }
                      frame 4 {
                        n563 = local write "Middle Finger"(TRUE ("Thumb 3")) -> ()
                        n564 = local write "Little Finger"(TRUE ("Thumb 5")) -> ()
                        n565 = local write "Ring Finger"(TRUE ("Thumb 4")) -> ()
                        n566 = local write "Index Finger"(TRUE ("Thumb 2")) -> ()
                      }
                    }
                    n567 = Add(x=w413, y=w414) -> (x+y=w415:dbl)
                    n568 = local write "Total Number of Fingers"(w415) -> ()
                    n569 = local write "Thumb"(w409) -> ()
                  }
                  n570 = local read "i"() -> (w405:i32)
                  n571 = Add(x=w405, y=1) -> (x+y=w407:i32)
                  n572 = local write "i"(w407) -> ()
                  n573 = local write "j"(0 ("j")) -> ()
                }
                n574 = local write "i"(0 ("i")) -> ()
                n575 = local write "j"(0 ("j")) -> ()
                n576 = local write "range"(230 ("range")) -> ()
              }
            }
            n577 = case shown="True" w328 {
              tunnel: w325 -> [_ w474]
              frame False {
              }
              frame True {
                # "hand from left"
                n578 = for {
                  tunnel: w474 -> [w479] mode=indexing
                  n579 = for {
                    tunnel: w479 -> [w512] mode=indexing
                    # "based on the number of fingers,\ndecide which led light is on"
                    # "if the thumb is on, the total number of finger +1"
                    # "within the threshold, if there is a black pixel, thumb counter +1"
                    n580 = local read "j"() -> (w508:i32)
                    n581 = call "BW-convert.vi"("Input pixel"=w512) -> ("Output pixel"=w494:dbl)  [unwired: 10 in]
                    n582 = Add(x=w508, y=1) -> (x+y=w509:i32)
                    n583 = local read "found fingers"() -> (w490:bool)
                    n584 = local write "j"(w509) -> ()
                    n585 = Not Equal?(x=w494, y=255.0) -> (x != y?=w498:bool)
                    n586 = local read "found fingers"() -> (w496:bool)
                    n587 = local read "range"() -> (w487:i32)
                    n588 = Equal?(x=w494, y=255.0) -> (x = y?=w491:bool)
                    n589 = local read "j"() -> (w499:i32)
                    n590 = local read "i"() -> (w505:i32)
                    n591 = local read "j"() -> (w502:i32)
                    n592 = Not(x=w496) -> (.not. x?=w495:bool)
                    n593 = Less Or Equal?(x=w502, y=170) -> (x <= y?=w500:bool)
                    n594 = Less Or Equal?(x=w505, y=110) -> (x <= y?=w503:bool)
                    n595 = Equal?(x=w499, y=w487) -> (x = y?=w492:bool)
                    n596 = Compound Arithmetic op=AND(w492, w491, w490) -> (w489:bool)
                    n597 = Compound Arithmetic op=AND(w498, w503, w500) -> (w506:bool)
                    n598 = Compound Arithmetic op=AND(w498, w492, w495) -> (w497:bool)
                    n599 = case shown="True" w506 {
                      frame False {
                      }
                      frame True {
                        n600 = local read "thumb counter"() -> (w542:i32)
                        n601 = Add(x=w542, y=1) -> (x+y=w540:i32)
                        n602 = local write "thumb counter"(w540) -> ()
                      }
                    }
                    n603 = case shown="True" w489 {
                      frame False {
                      }
                      frame True {
                        # "change the found fingers flag if there is a white pixel"
                        n604 = local write "found fingers"(FALSE ("found fingers")) -> ()
                      }
                    }
                    n605 = case shown="True" w497 {
                      frame False {
                      }
                      frame True {
                        # "count the total number of fingers (except thumb)"
                        n606 = local read "fingers counter"() -> (w538:i32)
                        n607 = local write "found fingers"(TRUE ("found fingers")) -> ()
                        n608 = Add(x=w538, y=1) -> (x+y=w537:i32)
                        n609 = local write "fingers counter"(w537) -> ()
                      }
                    }
                    n610 = local read "thumb counter"() -> (w510:i32)
                    n611 = Greater?(x=w510, y=100.0) -> (0:w488:bool)
                    n612 = local read "fingers counter"() -> (w486:i32)
                    n613 = local read "Thumb"() -> (w485:bool)
                    n614 = local read "fingers counter"() -> (w482:i32)
                    n615 = Select(t=1.0, s=w485, f=0.0) -> (s? t:f=w481:dbl)
                    n616 = case shown="3" w486 {
                      frame 0, Default {
                        n617 = local write "Middle Finger"(FALSE ("Thumb 3")) -> ()
                        n618 = local write "Little Finger"(FALSE ("Thumb 5")) -> ()
                        n619 = local write "Ring Finger"(FALSE ("Thumb 4")) -> ()
                        n620 = local write "Index Finger"(FALSE ("Thumb 2")) -> ()
                      }
                      frame 1 {
                        n621 = local write "Middle Finger"(FALSE ("Thumb 3")) -> ()
                        n622 = local write "Little Finger"(FALSE ("Thumb 5")) -> ()
                        n623 = local write "Ring Finger"(FALSE ("Thumb 4")) -> ()
                        n624 = local write "Index Finger"(TRUE ("Thumb 2")) -> ()
                      }
                      frame 2 {
                        n625 = local write "Middle Finger"(TRUE ("Thumb 3")) -> ()
                        n626 = local write "Little Finger"(FALSE ("Thumb 5")) -> ()
                        n627 = local write "Ring Finger"(FALSE ("Thumb 4")) -> ()
                        n628 = local write "Index Finger"(TRUE ("Thumb 2")) -> ()
                      }
                      frame 3 {
                        n629 = local write "Middle Finger"(TRUE ("Thumb 3")) -> ()
                        n630 = local write "Little Finger"(FALSE ("Thumb 5")) -> ()
                        n631 = local write "Ring Finger"(TRUE ("Thumb 4")) -> ()
                        n632 = local write "Index Finger"(TRUE ("Thumb 2")) -> ()
                        n633 = local write "range"(245 ("range")) -> ()
                      }
                      frame 4 {
                        n634 = local write "Middle Finger"(TRUE ("Thumb 3")) -> ()
                        n635 = local write "Little Finger"(TRUE ("Thumb 5")) -> ()
                        n636 = local write "Ring Finger"(TRUE ("Thumb 4")) -> ()
                        n637 = local write "Index Finger"(TRUE ("Thumb 2")) -> ()
                      }
                    }
                    n638 = local write "Thumb"(w488) -> ()
                    n639 = Add(x=w482, y=w481) -> (x+y=w480:dbl)
                    n640 = local write "Total Number of Fingers"(w480) -> ()
                  }
                  n641 = local read "i"() -> (w475:i32)
                  n642 = Add(x=w475, y=1) -> (x+y=w477:i32)
                  n643 = local write "i"(w477) -> ()
                  n644 = local write "j"(0 ("j")) -> ()
                }
                n645 = local write "i"(0 ("i")) -> ()
                n646 = local write "j"(0 ("j")) -> ()
                n647 = local write "range"(250 ("range")) -> ()
              }
            }
          }
        }
        n648 = local write "found fingers"(FALSE ("found fingers")) -> ()
      }
      event "Left": Value Change {
        n649 = event-data() -> ()  [unwired: 1 in, 6 out]
      }
      event "stop": Value Change {
        n650 = event-data() -> ()  [unwired: 1 in, 6 out]
      }
    }
    n651 = Or(x=w2, y="stop") -> (x .or. y?=w3:bool)
  }
  n652 = local write "Total Number of Fingers"(0 ("Total number of finger")) -> ()
